vi "Delete Product.vi"(8 "error in (no error)":errorcluster, 11 "Name":string) -> (0 "error out":errorcluster)   [LabVIEW 2020, in "SQLITE Inventory.lvlib"]
uses:
  SQLITE Inventory.lvlib
  <vilib>/drjdpowell/SQLite Library/SQL Connection/Open (path).vi
  <vilib>/drjdpowell/SQLite Library/SQL Connection/Open (string).vi
  <vilib>/AdvancedString/Path To Command Line String.vi
  <vilib>/drjdpowell/SQLite Library/SQL Connection/Execute SQL (No results).vi
  <vilib>/drjdpowell/SQLite Library/SQL Connection/Connection.lvclass
  <vilib>/drjdpowell/SQLite Library/SQLite.lvlib
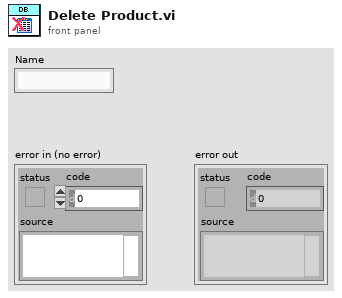
[diagram p1: front panel]
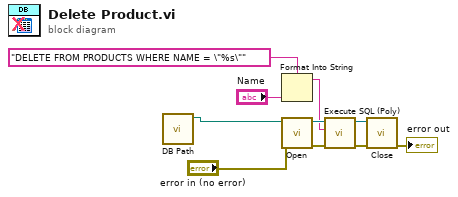
[diagram p0: block diagram]
diagram:
  n1 = call "DB Path.vi"() -> ("DB Path"=w3:path)  [unwired: 11 in]
  n2 = Format Into String(format string="DELETE FROM PRODUCTS WHERE NAME = \"%s\"", "Name") -> (resulting string=w4:string)  [unwired: 2 in, 1 out]
  n3 = call-poly <vilib>:"Open.vi"("error in (no error)"="error in (no error)", "db file"=w3) -> ("error out"=w7:errorcluster, "SQLite Connection"=w10:refnum<class "Connection.lvclass">)  [unwired: 8 in]
  n4 = call-poly <vilib>:"Execute SQL (Poly).vi"("error in (no error)"=w7, "SQL"=w4, "SQLite Connection in"=w10) -> ("error out"=w8:errorcluster, "SQLite Connection"=w9:refnum<class "Connection.lvclass">)  [unwired: 7 in]
  n5 = call-dynamic "Close.vi"("error in (no error)"=w8, "SQLite Connection in"=w9) -> ("error out"=→"error out":errorcluster)  [unwired: 9 in]
